vi "Periodic Tasks.vi"(8 "error in":errorcluster) -> ()   [LabVIEW 2013]
doc: "This VI runs in parallel to other tasks. It can contain as many user-defined periodic loops as you need. These can carry out PID or other sorts of timed response."
uses:
  <vilib>/Rock Robotics/SystemInterfaces/Utilities/FPGA_UtilitiesLED Source.ctl
  <vilib>/Rock Robotics/SystemInterfaces/Utilities/FPGA_UtilitiesLED State.ctl
  <vilib>/Rock Robotics/WPI/Compressor/WPI_CompressorGetSetRefNum.vi
  Robot Global Data.vi
  <vilib>/Rock Robotics/WPI/Solenoid/WPI_SolenoidValue.ctl
  <vilib>/Rock Robotics/WPI/Solenoid/WPI_SolenoidSetEnum.vi
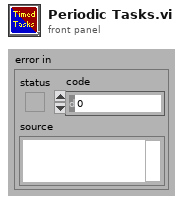
[diagram p1: front panel]
types:
  T1 = typedef "WPI_SolenoidValue.ctl" = enum16{"Off", "On", "Forward", "Reverse"}
  T2 = typedef "WPI_JoystickDevRef.ctl" = cluster{"Device":T3}
  T3 = typedef "WPI_JoystickDeviceEnum.ctl" = enum16{"USB 1", "USB 2", "USB 3", "USB 4", "Kinect 1", "Kinect 2"}
  T4 = typedef "WPI_SolenoidDevRef.ctl" = cluster{"DevStatus":errorcluster, "Solenoid Module":T5, "Forward Solenoid Channel":T6, "Reverse Solenoid Channel":T6}
  T5 = typedef "FPGA_TypedefSolenoidModule.ctl" = enum16{"Solenoid Module 1", "Solenoid Module 2"}
  T6 = typedef "WPI_SolenoidChannel.ctl" = enum8{"Solenoid 1", "Solenoid 2", "Solenoid 3", "Solenoid 4", "Solenoid 5", "Solenoid 6", "Solenoid 7", "Solenoid 8", "Invalid"}
  T7 = typedef "WPI_JoystickButtonState.ctl" = cluster{"Button 1":bool, "Button 2":bool, "Button 3":bool, "Button 4":bool, "Button 5":bool, "Button 6":bool, "Button 7":bool, "Button 8":bool, "Button 9":bool, "Button 10":bool, "Button 11":bool, "Button 12":bool}
  T8 = typedef "FPGA_UtilitiesLED State.ctl" = enum16{"Off", "On", "Toggle"}
  T9 = typedef "FPGA_UtilitiesLED Source.ctl" = enum16{"User LED", "FPGA LED"}
  T10 = typedef "WPI_CompressorDevRef.ctl" = cluster{"DevStatus":errorcluster, "DigitalInputDevRef":T11, "RelayDevRef":T14}
  T11 = typedef "WPI_DigitalInputDevRef.ctl" = cluster{"DevStatus":errorcluster, "DIO Channel":T12, "Digital Module":T13}
  T12 = typedef "FPGA_DIOChannel.ctl" = enum8{"DIO 1", "DIO 2", "DIO 3", "DIO 4", "DIO 5", "DIO 6", "DIO 7", "DIO 8", "DIO 9", "DIO 10", "DIO 11", "DIO 12", "DIO 13", "DIO 14", "Invalid"}
  T13 = typedef "FPGA_TypedefDigitalModule.ctl" = enum16{"Digital Module 1", "Digital Module 2"}
  T14 = typedef "WPI_RelayDevRef.ctl" = cluster{"DevStatus":errorcluster, "Relay Channel":T15, "Digital Module":T13, "Relay Direction":T16}
  T15 = typedef "FPGA_DIORelayChannel.ctl" = enum8{"Relay 1", "Relay 2", "Relay 3", "Relay 4", "Relay 5", "Relay 6", "Relay 7", "Relay 8", "Invalid"}
  T16 = typedef "WPI_RelayDirection.ctl" = enum16{"Both directions", "Forward only", "Reverse only"}
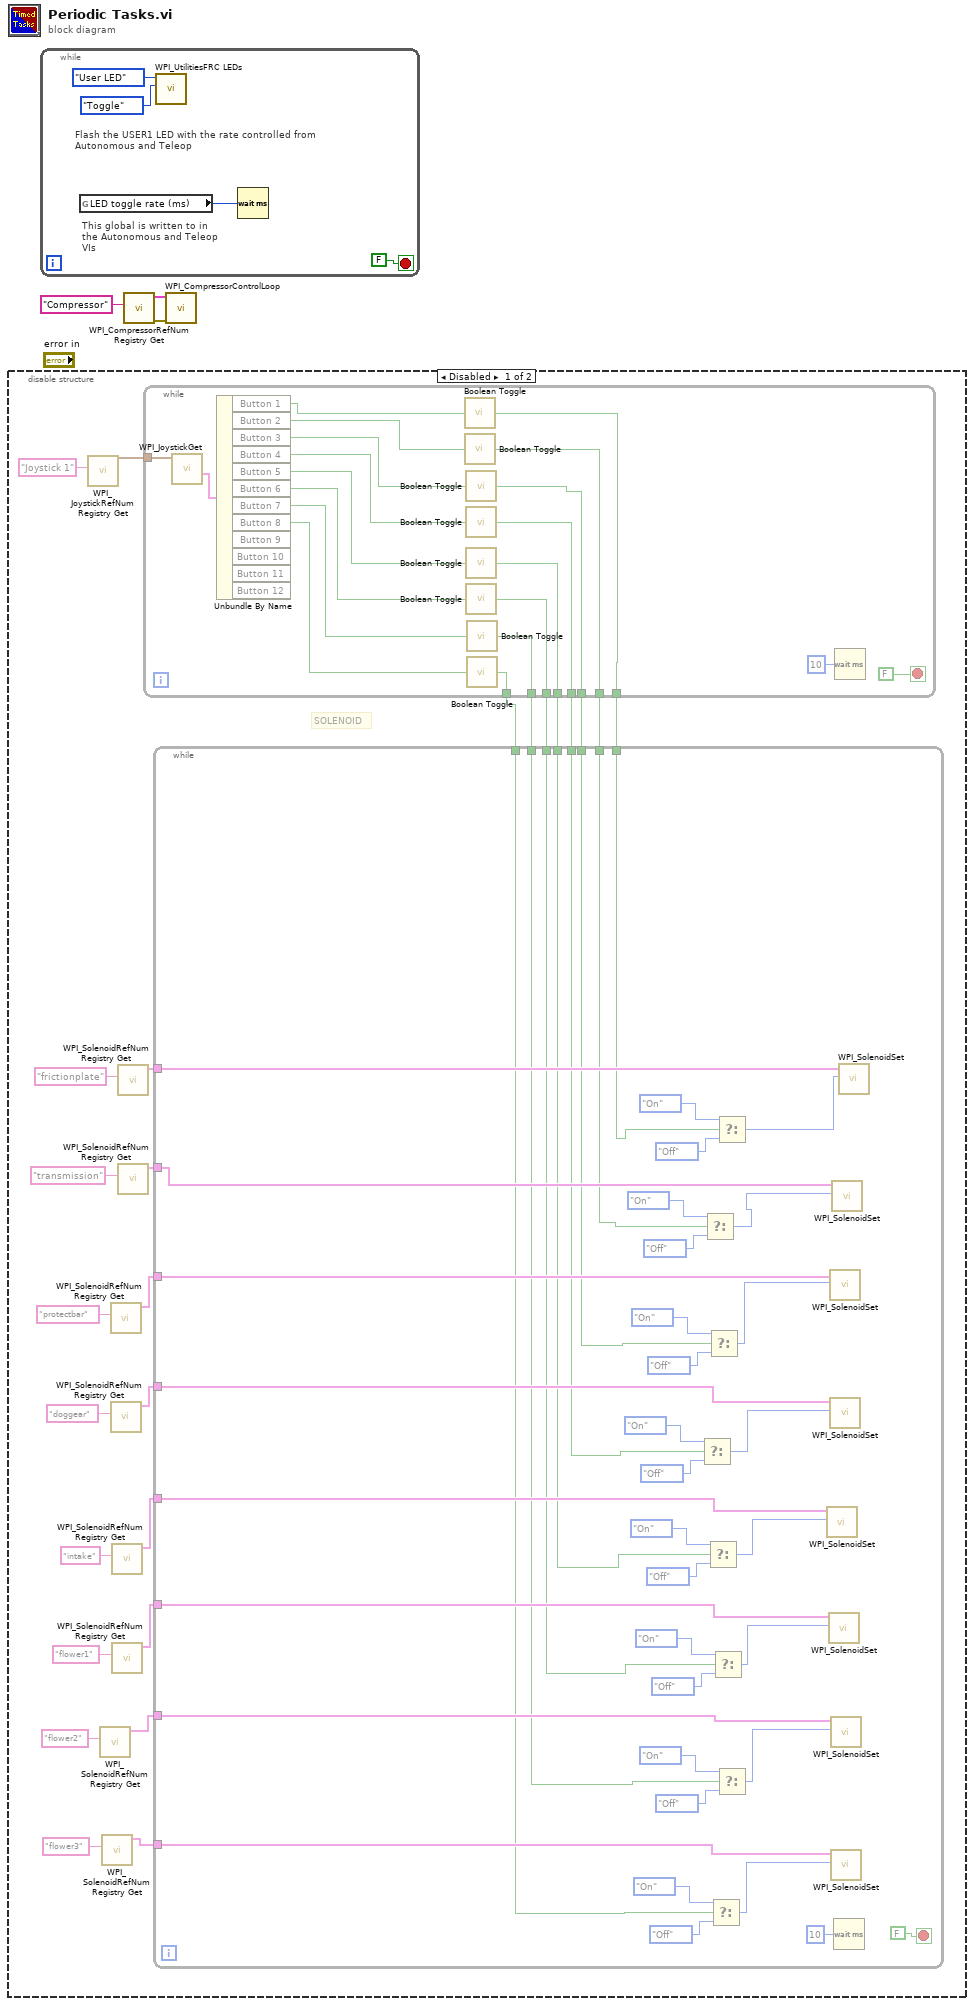
[diagram p0: block diagram]
diagram:
  n1 = disable-structure shown="Disabled" {
    frame Disabled {
      # "SOLENOID"
      n2 = call <vilib>:"WPI_JoystickRefNum Registry Get.vi"("refnum name"="Joystick 1") -> ("JoystickDevRef"=w4:T2)  [unwired: 1 in, 9 out]
      n3 = call <vilib>:"WPI_SolenoidRefNum Registry Get.vi"("refnum name"="flower2") -> ("SolenoidDevRef"=w14:T4)  [unwired: 9 in, 1 out]
      n4 = call <vilib>:"WPI_SolenoidRefNum Registry Get.vi"("refnum name"="flower3") -> ("SolenoidDevRef"=w13:T4)  [unwired: 9 in, 1 out]
      n5 = call <vilib>:"WPI_SolenoidRefNum Registry Get.vi"("refnum name"="protectbar") -> ("SolenoidDevRef"=w18:T4)  [unwired: 9 in, 1 out]
      n6 = call <vilib>:"WPI_SolenoidRefNum Registry Get.vi"("refnum name"="doggear") -> ("SolenoidDevRef"=w17:T4)  [unwired: 9 in, 1 out]
      n7 = call <vilib>:"WPI_SolenoidRefNum Registry Get.vi"("refnum name"="intake") -> ("SolenoidDevRef"=w16:T4)  [unwired: 9 in, 1 out]
      n8 = call <vilib>:"WPI_SolenoidRefNum Registry Get.vi"("refnum name"="flower1") -> ("SolenoidDevRef"=w15:T4)  [unwired: 9 in, 1 out]
      n9 = call <vilib>:"WPI_SolenoidRefNum Registry Get.vi"("refnum name"="frictionplate") -> ("SolenoidDevRef"=w25:T4)  [unwired: 9 in, 1 out]
      n10 = call <vilib>:"WPI_SolenoidRefNum Registry Get.vi"("refnum name"="transmission") -> ("SolenoidDevRef"=w27:T4)  [unwired: 9 in, 1 out]
      n11 = while {
        tunnel: [w39] -> w12
        tunnel: [w38] -> w11
        tunnel: [w37] -> w10
        tunnel: [w36] -> w9
        tunnel: [w35] -> w8
        tunnel: [w34] -> w7
        tunnel: [w33] -> w6
        tunnel: [w32] -> w5
        tunnel: w4 -> [w30]
        stop <- FALSE stop-if-true
        n12 = call <vilib>:"WPI_JoystickGet.vi"("JoystickDevRef"=w30) -> ("Buttons"=w47:T7)  [unwired: 4 in, 2 out]
        n13 = Unbundle By Name(w47) -> ("Button 1"=w31:bool, "Button 2"=w46:bool, "Button 3"=w45:bool, "Button 4"=w44:bool, "Button 5"=w43:bool, "Button 6"=w42:bool, "Button 7"=w41:bool, "Button 8"=w40:bool)  [unwired: 4 out]
        n14 = call "Boolean Toggle.vi"("Input"=w31) -> ("Output"=w32:bool)
        n15 = call "Boolean Toggle.vi"("Input"=w46) -> ("Output"=w33:bool)
        n16 = call "Boolean Toggle.vi"("Input"=w45) -> ("Output"=w34:bool)
        n17 = call "Boolean Toggle.vi"("Input"=w44) -> ("Output"=w35:bool)
        n18 = call "Boolean Toggle.vi"("Input"=w43) -> ("Output"=w36:bool)
        n19 = call "Boolean Toggle.vi"("Input"=w42) -> ("Output"=w37:bool)
        n20 = call "Boolean Toggle.vi"("Input"=w41) -> ("Output"=w38:bool)
        n21 = call "Boolean Toggle.vi"("Input"=w40) -> ("Output"=w39:bool)
        n22 = Wait (ms)(milliseconds to wait=u32 10) -> ()  [unwired: 1 out]
      }
      n23 = while {
        tunnel: w27 -> [w89]
        tunnel: w25 -> [w90]
        tunnel: w18 -> [w88]
        tunnel: w17 -> [w87]
        tunnel: w16 -> [w86]
        tunnel: w15 -> [w85]
        tunnel: w14 -> [w84]
        tunnel: w13 -> [w83]
        tunnel: w12 -> [w58]
        tunnel: w11 -> [w57]
        tunnel: w10 -> [w56]
        tunnel: w9 -> [w55]
        tunnel: w8 -> [w54]
        tunnel: w7 -> [w53]
        tunnel: w6 -> [w52]
        tunnel: w5 -> [w51]
        stop <- FALSE stop-if-true
        n24 = Select(t=WPI_SolenoidValue."On" ("Value"), s=w54, f=WPI_SolenoidValue."Off" ("Value")) -> (s? t:f=w61:T1)
        n25 = Select(t=WPI_SolenoidValue."On" ("Value"), s=w52, f=WPI_SolenoidValue."Off" ("Value")) -> (s? t:f=w59:T1)
        n26 = Select(t=WPI_SolenoidValue."On" ("Value"), s=w55, f=WPI_SolenoidValue."Off" ("Value")) -> (s? t:f=w62:T1)
        n27 = Select(t=WPI_SolenoidValue."On" ("Value"), s=w53, f=WPI_SolenoidValue."Off" ("Value")) -> (s? t:f=w60:T1)
        n28 = Select(t=WPI_SolenoidValue."On" ("Value"), s=w58, f=WPI_SolenoidValue."Off" ("Value")) -> (s? t:f=w65:T1)
        n29 = Select(t=WPI_SolenoidValue."On" ("Value"), s=w56, f=WPI_SolenoidValue."Off" ("Value")) -> (s? t:f=w63:T1)
        n30 = Select(t=WPI_SolenoidValue."On" ("Value"), s=w51, f=WPI_SolenoidValue."Off" ("Value")) -> (s? t:f=w80:T1)
        n31 = Select(t=WPI_SolenoidValue."On" ("Value"), s=w57, f=WPI_SolenoidValue."Off" ("Value")) -> (s? t:f=w64:T1)
        n32 = call-poly <vilib>:"WPI_SolenoidSet.vi"("Value"=w62, "SolenoidDevRef"=w86) -> ()  [unwired: 8 in, 2 out]
        n33 = call-poly <vilib>:"WPI_SolenoidSet.vi"("Value"=w63, "SolenoidDevRef"=w85) -> ()  [unwired: 8 in, 2 out]
        n34 = call-poly <vilib>:"WPI_SolenoidSet.vi"("Value"=w60, "SolenoidDevRef"=w88) -> ()  [unwired: 8 in, 2 out]
        n35 = call-poly <vilib>:"WPI_SolenoidSet.vi"("Value"=w61, "SolenoidDevRef"=w87) -> ()  [unwired: 8 in, 2 out]
        n36 = call-poly <vilib>:"WPI_SolenoidSet.vi"("Value"=w64, "SolenoidDevRef"=w84) -> ()  [unwired: 8 in, 2 out]
        n37 = call-poly <vilib>:"WPI_SolenoidSet.vi"("Value"=w65, "SolenoidDevRef"=w83) -> ()  [unwired: 8 in, 2 out]
        n38 = call-poly <vilib>:"WPI_SolenoidSet.vi"("Value"=w59, "SolenoidDevRef"=w89) -> ()  [unwired: 8 in, 2 out]
        n39 = Wait (ms)(milliseconds to wait=u32 10) -> ()  [unwired: 1 out]
        n40 = call-poly <vilib>:"WPI_SolenoidSet.vi"("Value"=w80, "SolenoidDevRef"=w90) -> ()  [unwired: 8 in, 2 out]
      }
    }
    frame Enabled {
    }
  }
  n41 = while {
    stop <- FALSE stop-if-true
    # "This global is written to in the Autonomous and Teleop VIs"
    # "Flash the USER1 LED with the rate controlled from Autonomous and Teleop"
    n42 = global read "Robot Global Data.vi" "LED toggle rate (ms)"() -> (w92:u32)
    n43 = call <vilib>:"WPI_UtilitiesFRC LEDs.vi"("State"=FPGA_UtilitiesLED_State."Toggle", "LED Type"=FPGA_UtilitiesLED_Source."User LED") -> ()  [unwired: 1 in, 9 out]
    n44 = Wait (ms)(milliseconds to wait=w92) -> ()  [unwired: 1 out]
  }
  n45 = call <vilib>:"WPI_CompressorRefNum Registry Get.vi"("refnum name"="Compressor") -> ("error out"=w2:errorcluster, "CompressorDevRef"=w3:T10)  [unwired: 9 in]
  n46 = call <vilib>:"WPI_CompressorControlLoop.vi"("error in (no error)"=w2, "CompressorDevRef"=w3) -> ()  [unwired: 10 in]
